vi "DrawVerticalLineOnGraph (SubVI).vi"(2 "Array":dbl[](array[numeric]), 3 "value uncertainty":dbl, 4 "x = value":dbl) -> (0 "X error bars":cluster{dbl[], dbl[]}(graph), 1 "Line at x = value":cluster{dbl[], dbl[]})   [LabVIEW 2016]
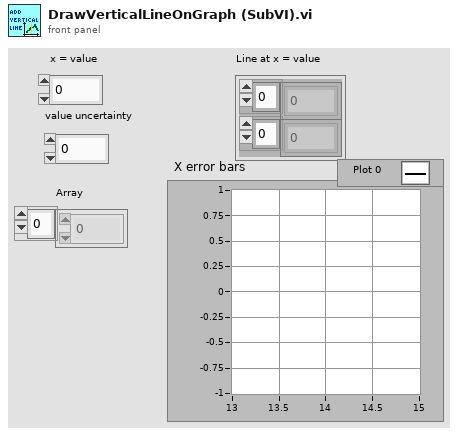
[diagram p1: front panel]
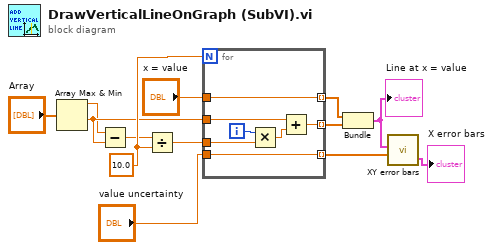
[diagram p0: block diagram]
diagram:
  w13 = 10.0 ("y")
  n1 = Array Max & Min(array="Array") -> (max value=w8:dbl, min value=w11:dbl)  [unwired: 2 out]
  n2 = Subtract(x=w8, y=w11) -> (x-y=w9:dbl)
  n3 = Divide(x=w9, y=w13) -> (x/y=w10:dbl)
  n4 = for {
    N: w13 -> [_]
    tunnel: w11 -> [w20]
    tunnel: [w19] -> w12 mode=indexing
    tunnel: w10 -> [w17]
    tunnel: [w15] -> w6 mode=indexing
    tunnel: "x = value" -> [w15]
    tunnel: "value uncertainty" -> [w14]
    tunnel: [w14] -> w3 mode=indexing
    i -> [w18]
    n5 = Multiply(x=w18, y=w17) -> (x*y=w16:dbl)
    n6 = Add(x=w20, y=w16) -> (x+y=w19:dbl)
  }
  n7 = Bundle(w6, w12) -> (w2:cluster{dbl[], dbl[]})  [unwired: 1 in]
  "Line at x = value" <- w2
  n8 = call "XY error bars.vi"("XY plot"=w2, "Xerror"=w3) -> ("X error bars"=→"X error bars":cluster{dbl[], dbl[]})  [unwired: 6 in, 2 out]
